vi "Run Project Unit Tests.vi"(6 "Variant in":variant, 7 "Shift Pressed?":bool, 8 "error in (no error)":errorcluster, 10 "QD Combo Box Ref":refnum<vi>, 11 "QD Launch VI Ref":refnum<vi>) -> (0 "error out":errorcluster, 4 "Variant out":variant)   [LabVIEW 2013]
doc: "This QD shortcut will discover all the Caraya Unit Tests in a project and run them in interactive mode.\n\nDefault Shortcut - [U]"
uses:
  classes/Test Runner/Test Runner.lvclass/Test Runner.ctl
  classes/Test Runner.Project/Test Runner.Project.lvclass/Test Runner.Project.ctl
  classes/Test Runner.Project/Test Runner.Project.lvclass
  classes/Test Runner/Test Runner.lvclass
panel:
  out "Virtual Folder":string
  out "Test VIs":path[](array[path])
  in  "Undo Name":string="Run Project Unit Tests"
  # "Do not change the connector pane of this VI.\n\nSee the block diagram for directions on how to use this template."
  # "Specify the name of the Undo transaction"
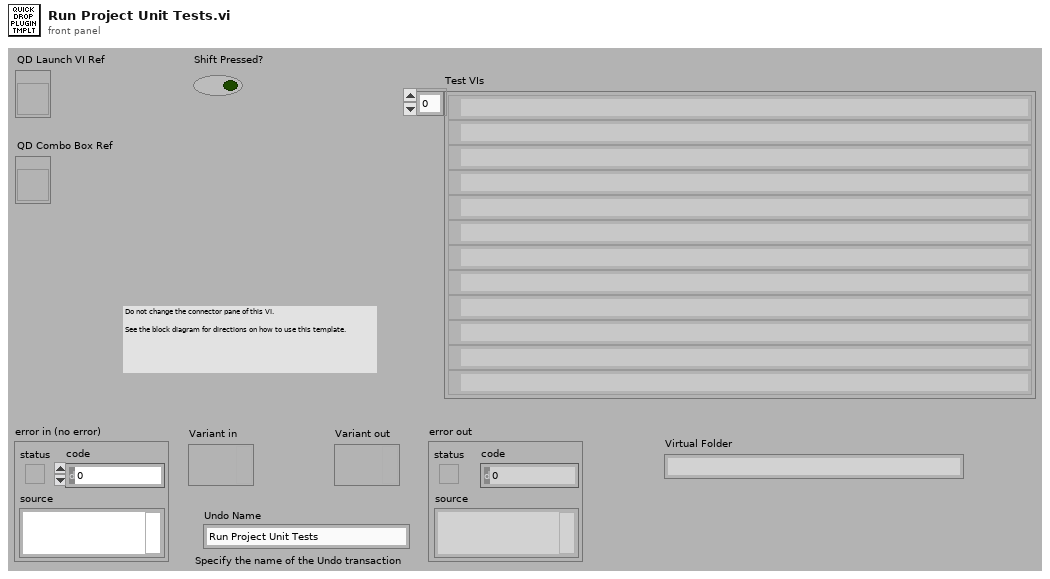
[diagram p1: front panel]
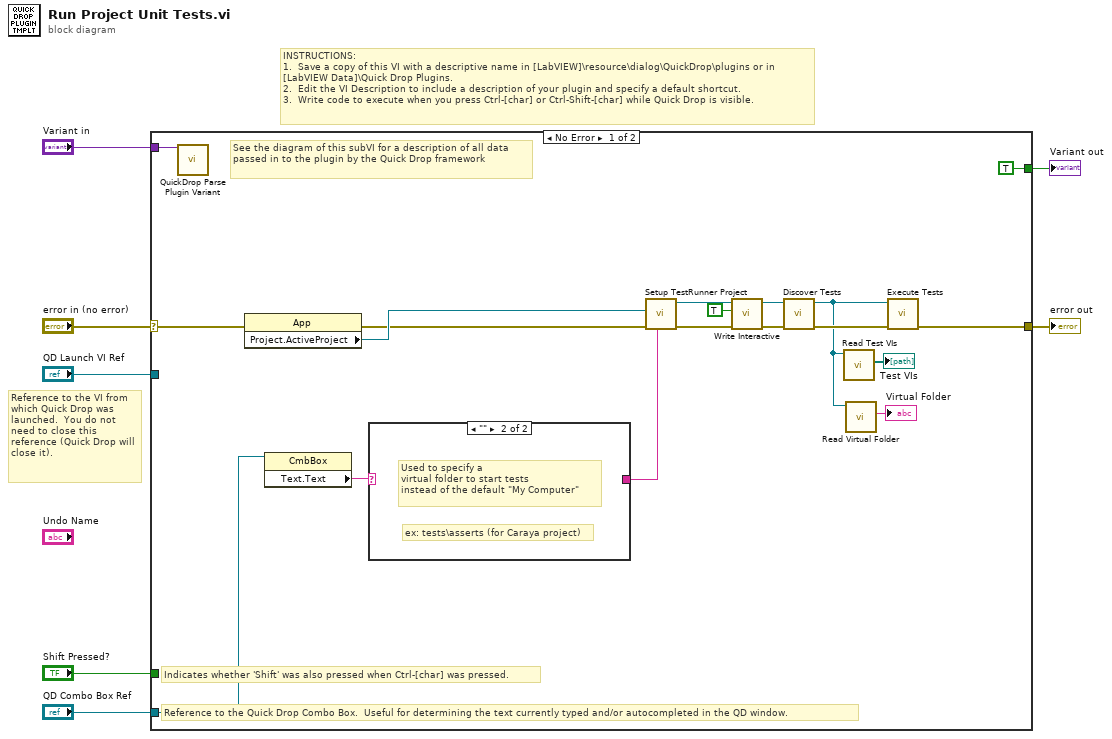
[diagram p0: block diagram]
diagram:
  # "Reference to the VI from which Quick Drop was launched.  You do not need to close this reference (Quick Drop will close it)."
  # "INSTRUCTIONS:\n1.  Save a copy of this VI with a descriptive name in [LabVIEW]\\resource\\dialog\\QuickDrop\\plugins or in [LabVIEW Data]\\Quick Drop Plugins.\n2.  Edit the VI Description to include a description of your plugin and specify a default shortcut. \n3.  Write code to execute when you press Ctrl-[char] or Ctrl-Shift-[char] while Quick Drop is visible."
  n1 = case shown="No Error" "error in (no error)" {
    selector: "error in (no error)" -> [w18 w26]
    tunnel: [w19 w26] -> w6
    tunnel: "QD Launch VI Ref" -> [_ _]
    tunnel: "Shift Pressed?" -> [_ _]
    tunnel: "QD Combo Box Ref" -> [w16 _]
    tunnel: "Variant in" -> [w24 _]
    tunnel: [TRUE _] -> w1
    frame No Error {
      # "See the diagram of this subVI for a description of all data passed in to the plugin by the Quick Drop framework"
      # "Reference to the Quick Drop Combo Box.  Useful for determining the text currently typed and/or autocompleted in the QD window."
      # "Indicates whether 'Shift' was also pressed when Ctrl-[char] was pressed."
      n2 = call <vilib>:"QuickDrop Parse Plugin Variant.vi"("QDKS Variant in"=w24) -> ()  [unwired: 12 in, 3 out]
      n3 = property on="Property Node" class="App"(error in=w18) -> (error out=w17:errorcluster, "Project.ActiveProject"=w22:refnum<vi>)  [unwired: 1 in, 1 out]
      n4 = property on="Property Node" class="CmbBox"(reference=w16) -> ("Text.Text"=w15:string)  [unwired: 1 in, 2 out]
      n5 = case shown="\"\"" w15 {
        selector: w15 -> [w25 _]
        tunnel: [w25 _] -> w8
        frame Default {
        }
        frame "" {
          # "ex: tests\\asserts (for Caraya project)"
          # "Used to specify a\nvirtual folder to start tests\ninstead of the default \"My Computer\""
        }
      }
      n6 = call "Setup TestRunner Project.vi"("Virtual Folder (empty: \"My Computer\")"=w8, "error in (no error)"=w17, "Project Refnum"=w22) -> ("error out"=w21:errorcluster, "Test Runner.Project out"=w13:refnum<class "Test Runner.Project.lvclass">)  [unwired: 7 in]
      n7 = call "Write Interactive.vi"("Interactive"=TRUE, "Test Runner in"=w13) -> ("Test Runner out"=w12:refnum<class "Test Runner.Project.lvclass">)  [unwired: 9 in]
      n8 = call "Discover Tests.vi"("error in (no error)"=w21, "Test Runner in"=w12) -> ("error out"=w20:errorcluster, "Test Runner out"=w10:refnum<class "Test Runner.Project.lvclass">)  [unwired: 8 in]
      n9 = call-dynamic "Read Test VIs.vi"("Test Runner in"=w10) -> ("Test VIs"=→"Test VIs":path[])  [unwired: 8 in, 2 out]
      n10 = call "Read Virtual Folder.vi"("Test Runner.Project in"=w10) -> ("Virtual Folder"=→"Virtual Folder":string)  [unwired: 9 in, 1 out]
      n11 = call-dynamic "Execute Tests.vi"("error in (no error)"=w20, "Test Runner in"=w10) -> ("error out"=w19:errorcluster)  [unwired: 8 in, 1 out]
    }
    frame Error {
    }
  }
  "error out" <- w6
  "Variant out" <- w1
